vi "Parameter Set Write Array.vi"(8 "error in":errorcluster, 10 "Control Mode STS":i32[](array[numeric]), 11 "Parameter Set in":refnum<class "Parameter Set.lvclass">) -> (0 "error out":errorcluster, 3 "Parameter Set out":refnum<class "Parameter Set.lvclass">)   [LabVIEW 2023, in "Parameter Set.lvclass"]
uses:
  Parameter Set.lvclass
  Parameter Set.lvclass/Parameter Set.ctl
  <vilib>/ADAS Replay HIL/Channels/Tag Wrapper/Polymorphic/Write Channel (I32).vi
  <vilib>/ADAS Replay HIL/Channels/Tag Wrapper/Polymorphic/Write Channel (I32).vi/cccb8e89-591f-4bb4-9d4e-ae06ba1f5498.vi
  <vilib>/ADAS Replay HIL/Channels/Tag Wrapper/Polymorphic/Write Channel (I32).vi/cccb8e89-591f-4bb4-9d4e-ae06ba1f5498.vi/4bc1c15b-36ab-481f-b8dd-c64075ce723a.vi
  <vilib>/ADAS Replay HIL/Channels/Tag Wrapper/Polymorphic/Write Channel (I32).vi/cccb8e89-591f-4bb4-9d4e-ae06ba1f5498.vi/d83cb72b-7713-41fc-a3d1-682de79cf574.vi
  <vilib>/ADAS Replay HIL/Channels/Tag Wrapper/Tag Wrapper.lvlib
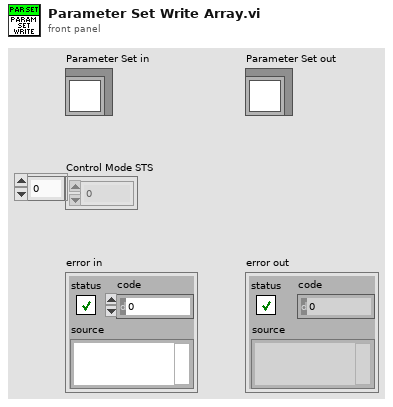
[diagram p1: front panel]
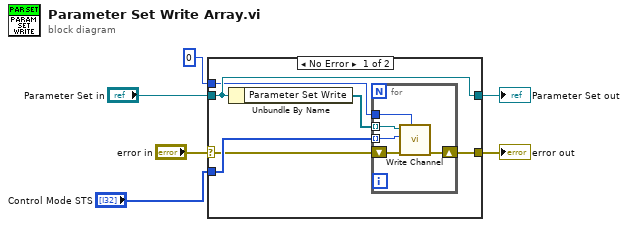
[diagram p0: block diagram]
diagram:
  n1 = case shown="No Error" "error in" {
    selector: "error in" -> [w9 w19]
    tunnel: [w8 w19] -> w5
    tunnel: [w11 w18] -> w3
    tunnel: "Parameter Set in" -> [w11 w18]
    tunnel: "Control Mode STS" -> [w10 _]
    tunnel: 0 ("Timeout (ms)") -> [w7 _]
    frame No Error {
      n2 = Unbundle By Name(w11) -> ("Parameter Set Write"=w12:refnum<k21>[])
      n3 = for {
        shift-right: [w16] -> w8
        shift-left: w9 -> [w17]
        tunnel: w12 -> [w15] mode=indexing
        tunnel: w10 -> [w14] mode=indexing
        tunnel: w7 -> [w13]
        n4 = call-poly <vilib>:"Write Channel.vi"("Timeout (ms)"=w13, "error in"=w17, "Value to Write"=w14, "ADAS HIL Channel in"=w15) -> ("error out"=w16:errorcluster)  [unwired: 5 in, 2 out]
      }
    }
    frame Error {
    }
  }
  "error out" <- w5
  "Parameter Set out" <- w3
